vi "Place the centering dot.vi"(6 "Color":u32(colorbox)=16711680, 7 "Image IN":T1, 8 "y (R)":dbl, 9 "x (R)":dbl, 10 "y (L)":dbl, 11 "x (L)":dbl) -> (3 "Image OUT":T1)   [LabVIEW 2018]
uses:
  <vilib>/vision/Image Controls.llb/IMAQ Image.ctl
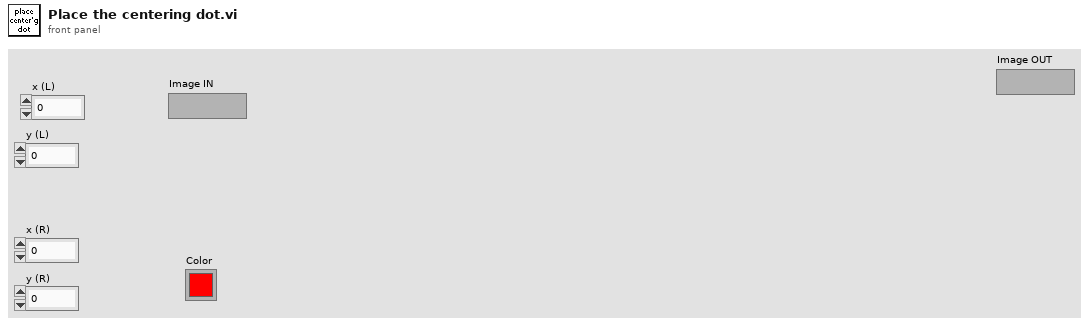
[diagram p1: front panel]
types:
  T1 = typedef "IMAQ Image.ctl" = refnum<image>
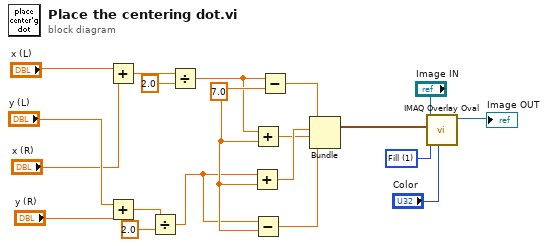
[diagram p0: block diagram]
diagram:
  w9 = u32 1 items=["Frame", "Fill"] ("Drawing Mode (Frame)")
  w19 = 7.0 ("y")
  n1 = Add(x="x (L)", y="x (R)") -> (x+y=w15:dbl)
  n2 = Add(x="y (L)", y="y (R)") -> (x+y=w11:dbl)
  n3 = Divide(x=w11, y=2.0) -> (x/y=w10:dbl)
  n4 = Divide(x=w15, y=2.0) -> (x/y=w13:dbl)
  n5 = Add(x=w10, y=w19) -> (x+y=w18:dbl)
  n6 = Add(x=w13, y=w19) -> (x+y=w17:dbl)
  n7 = Subtract(x=w10, y=w19) -> (x-y=w20:dbl)
  n8 = Subtract(x=w13, y=w19) -> (x-y=w16:dbl)
  n9 = Bundle(w16, w18, w17, w20) -> (w8:cluster{dbl, dbl, dbl, dbl})  [unwired: 1 in]
  n10 = call "IMAQ Overlay Oval"("Color"="Color", "Drawing Mode (Frame)"=w9, "Bounding Rectangle"=w8, "Image"="Image IN") -> ("Image Out"=→"Image OUT":T1)  [unwired: 6 in, 1 out]
